vi "GetWatchdogTimeouts.vi"(8 "error in (no error)":errorcluster) -> (0 "error out":errorcluster, 3 "software timeout":u32)   [LabVIEW 2017, in "GlobalConfiguration.lvlib"]
uses:
  <vilib>/addons/InsightCM/Utilities/GlobalConfiguration/GlobalConfiguration.lvlib
  <vilib>/addons/PointValueMap/subVIs/Point_Read_i32.vi
  <vilib>/addons/PointValueMap/PointValueMap.lvlib
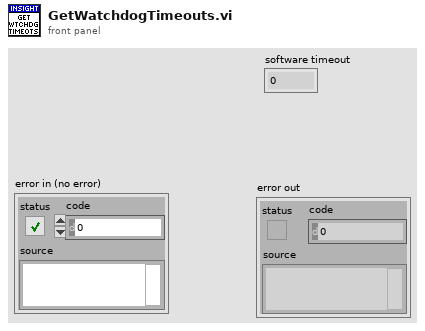
[diagram p1: front panel]
types:
  T1 = typedef "PointValueMap.lvlib/PointMap.ctl" = refnum<data-value>
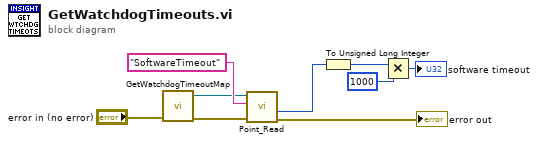
[diagram p0: block diagram]
diagram:
  n1 = call <vilib>:"GetWatchdogTimeoutMap.vi"("error in (no error)"="error in (no error)") -> ("error out"=w8:errorcluster, "WatchDogMap"=w6:T1)  [unwired: 9 in]
  n2 = call-poly <vilib>:"Point_Read.vi"("Error In"=w8, "Tag"="SoftwareTimeout", "Map"=w6) -> ("Error Out"=→"error out":errorcluster, "Value"=w5:i32)  [unwired: 3 in, 4 out]
  n3 = To Unsigned Long Integer(number=w5) -> (unsigned 32bit integer=w2:u32)
  n4 = Multiply(x=w2, y=u32 1000) -> (x*y=→"software timeout":u32)
